vi "Write Station status.vi"(7 "Send any changes now? (F)":bool, 8 "error in (no error)":errorcluster, 10 "Station status":T1, 11 "Fiber Auto Collimation state data in":refnum<class "Fiber Auto Collimation state data.lvclass">) -> (0 "error out":errorcluster, 3 "Fiber Auto Collimation state data out":refnum<class "Fiber Auto Collimation state data.lvclass">)   [LabVIEW 2018, in "Fiber Auto Collimation state data.lvclass"]
doc: "The main purpose of these states is to define the appearance (or lack thereof) of the main VI's front panel.\n\nThe default template is set up so that when \"Running\" the main window will be hidden, with asynchronous panels having been launched to handle all UI and other needs.\n\nIn the other states, the default template will be visible with a short message indicating the current status.\n\nThe above may change based on the needs of stations derived from the template, and other options may be added as well."
uses:
  Fiber Auto Collimation state data.lvclass
  Station status.ctl
  Fiber Auto Collimation state data.lvclass/Fiber Auto Collimation state data.ctl
  Tracked state data.ctl
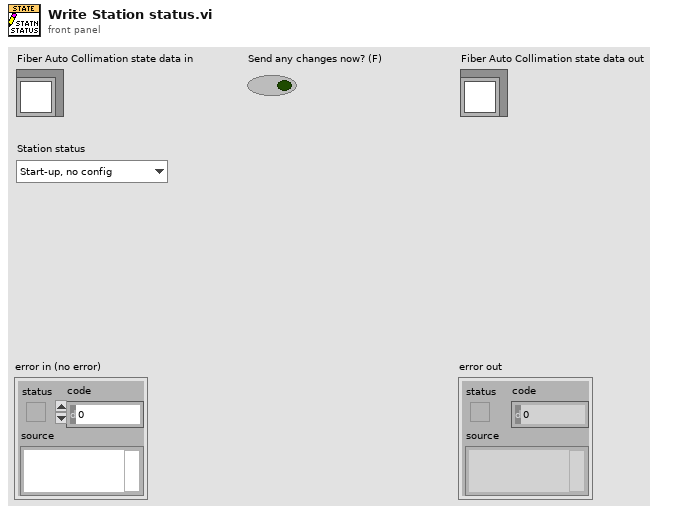
[diagram p1: front panel]
types:
  T1 = typedef "Fiber Auto Collimation state data.lvclass/Station status.ctl" = enum16{"Start-up, no config", "Start-up, config loaded", "Start-up, config problem", "Running", "Shutting down"}
  T2 = typedef "Fiber Auto Collimation state data.lvclass/Tracked state data.ctl" = enum16{"No update", "Permission level", "Username", "Test running", "DUT Serial", "Test status", "MOM Lot", "Loaded test recipe", "Model case running", "Station status", "BV data", "Defect Identify data", "Axis Position data", "Fiber Ass PN", "Operator", "RunTime", "VBAI", "Steps Cycle Time"}
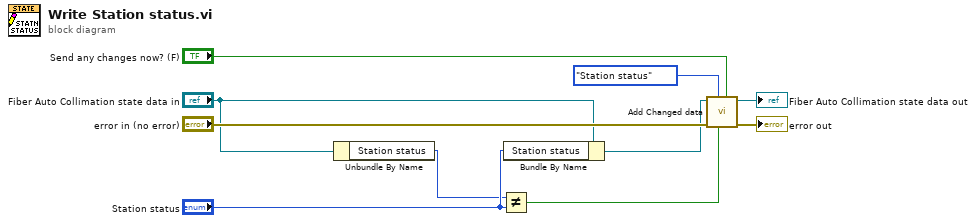
[diagram p0: block diagram]
diagram:
  n1 = Unbundle By Name("Fiber Auto Collimation state data in") -> ("Station status"=w2:T1)
  n2 = Not Equal?(x=w2, y="Station status") -> (x != y?=w3:bool)
  n3 = Bundle By Name(cluster="Fiber Auto Collimation state data in", "Station status"="Station status") -> (w6:refnum<class "Fiber Auto Collimation state data.lvclass">)
  n4 = call "Add Changed data.vi"("Send any changes now? (F)"="Send any changes now? (F)", "Data changed?"=w3, "Data type"=Tracked_state_data."Station status", "error in (no error)"="error in (no error)", "Fiber Auto Collimation state data in"=w6) -> ("error out"=→"error out":errorcluster, "Fiber Auto Collimation state data out"=→"Fiber Auto Collimation state data out":refnum<class "Fiber Auto Collimation state data.lvclass">)  [unwired: 5 in]
